vi "流程参数读取.vi"(7 "是否启用通讯通知":bool, 8 "error in (no error)":errorcluster, 11 "Slave ID":T2) -> (0 "error out":errorcluster, 3 "参数":T1)   [LabVIEW 2016, in "质控单元V1.lvlib"]
uses:
  <vilib>/Plasmionique/MB Master/MB_Master/MB_Master.lvclass
  <vilib>/Plasmionique/MB Master/MB Master.lvlib
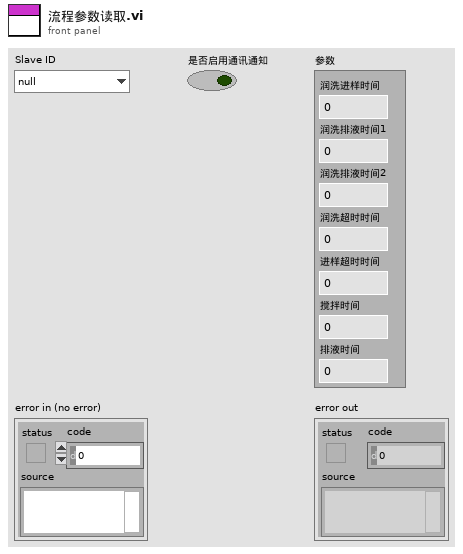
[diagram p1: front panel]
types:
  T1 = cluster{"润洗进样时间":sgl, "润洗排液时间1":sgl, "润洗排液时间2":sgl, "润洗超时时间":sgl, "进样超时时间":sgl, "搅拌时间":sgl, "排液时间":sgl}
  T2 = typedef "质控单元V1.lvlib/质控slave id.ctl" = enum16{"null", "氨氮", "总磷", "CODMn", "CODCr", "总氮"}
  T3 = cluster{"[0]":dbl, "[1]":dbl, "[2]":dbl, "[3]":dbl, "[4]":dbl, "[5]":dbl, "[6]":dbl}
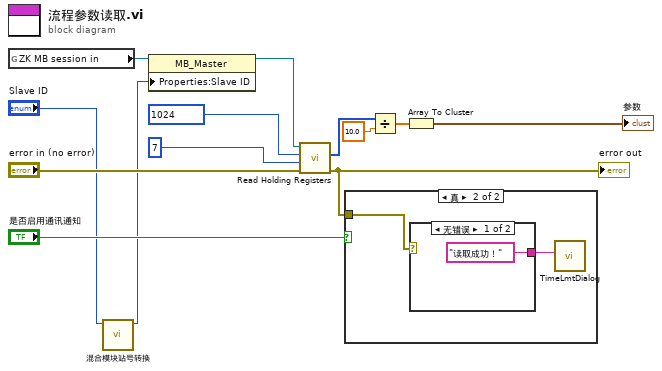
[diagram p0: block diagram]
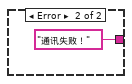
[diagram p3: hidden frame]
diagram:
  n1 = global read "ZK非断电保存全局变量.vi" "ZK MB session in"() -> (w12:refnum<class "MB_Master.lvclass">)
  n2 = call "混合模块站号转换.vi"("Slave ID输入"="Slave ID") -> ("Slave ID输出"=w1:T2)  [unwired: 10 in]
  n3 = property class="MB_Master"(reference=w12, "Properties:Slave ID"=w1) -> (reference out=w10:refnum<class "MB_Master.lvclass">)  [unwired: 1 in, 1 out]
  n4 = call <vilib>:"Read Holding Registers.vi"("error in (no error)"="error in (no error)", "quantity"=u16 7, "starting address"=u16 1024, "MB session in"=w10) -> ("error out"=w7:errorcluster, "Registers"=w3:u16[])  [unwired: 5 in, 1 out]
  "error out" <- w7
  n5 = case shown="真" "是否启用通讯通知" {
    tunnel: w7 -> [_ w15]
    frame False {
    }
    frame True {
      n6 = case shown="无错误" w15 {
        tunnel: ["读取成功！" "通讯失败！"] -> w14
        frame No Error {
        }
        frame Error {
        }
      }
      n7 = call "TimeLmtDialog.vi"("Infoin"=w14) -> ()  [unwired: 11 in]
    }
  }
  n8 = Divide(x=w3, y=10.0) -> (x/y=w5:dbl[])
  n9 = Array To Cluster(array=w5) -> (cluster=→"参数":T3)
